vi "subDFD_REMEZ Spec Conversion.vi"(6 "fs [Hz]":dbl=1.0, 7 "Filter Type":T2(ring), 8 "f4 [Hz]":dbl, 9 "f3 [Hz]":dbl, 10 "f2 [Hz]":dbl=0.45, 11 "f1 [Hz]":dbl=0.12) -> (2 "band specs":T1(array[cluster])=[{"band specification"=[{"freq"=0.0, "amplitude"=1.0, "weight"=1.0}, {"freq"=0.2, "amplitude"=1.0, "weight"=1.0}], "ripple constraint"=0.0}, {"band specification"=[{"freq"=0.3, "amplitude"=0.0, "weight"=1.0}, {"freq"=0.5, "amplitude"=0.0, "weight"=1.0}], "ripple constraint"=0.0}])   [LabVIEW 2023]
panel:
  # "freq"
  # "amplitude"
  # "weight"
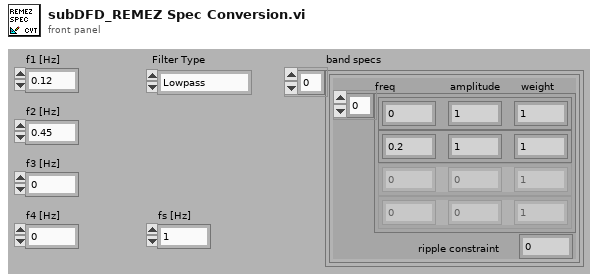
[diagram p1: front panel]
types:
  T1 = cluster{"band specification":cluster{"freq":dbl, "amplitude":dbl, "weight":dbl}[], "ripple constraint":dbl}[]
  T2 = enum16{"Lowpass", "Highpass", "Bandpass", "Bandstop"}
  T3 = cluster{cluster{"f2 [Hz]":dbl, dbl, dbl}[], dbl}[]
  T4 = cluster{cluster{"f4 [Hz]":dbl, dbl, dbl}[], dbl}[]
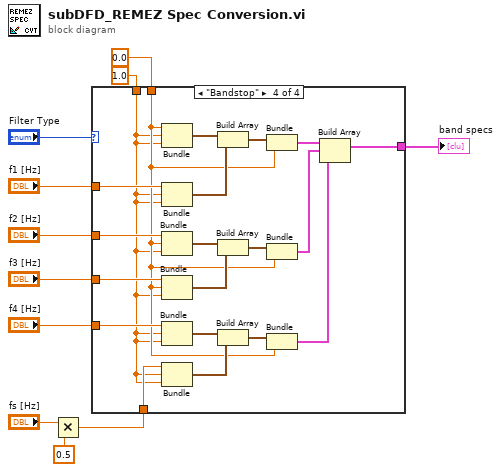
[diagram p0: block diagram]
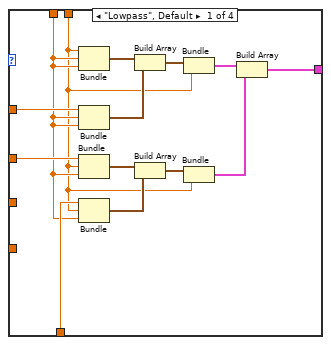
[diagram p2: hidden frame]
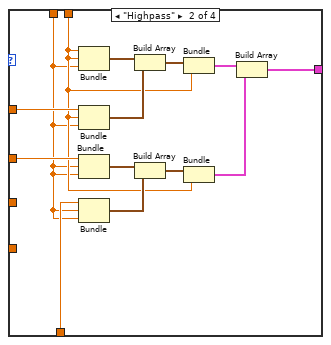
[diagram p3: hidden frame]
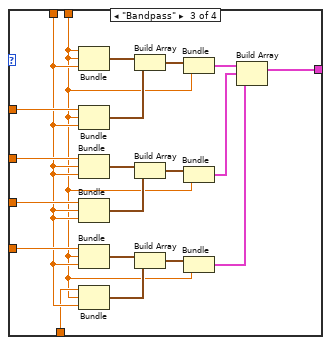
[diagram p4: hidden frame]
diagram:
  n1 = Multiply(x="fs [Hz]", y=0.5) -> (x*y=w4:dbl)
  n2 = case shown="\"Bandstop\"" "Filter Type" {
    tunnel: "f1 [Hz]" -> [w25 w39 w59 w79]
    tunnel: "f2 [Hz]" -> [w24 w38 w58 w78]
    tunnel: 0.0 -> [w15 w27 w42 w61]
    tunnel: 1.0 -> [w22 w26 w47 w60]
    tunnel: w4 -> [w23 w37 w46 w67]
    tunnel: [w12 w28 w40 w62] -> w3
    tunnel: "f3 [Hz]" -> [_ _ w49 w69]
    tunnel: "f4 [Hz]" -> [_ _ w48 w68]
    frame "Lowpass", Default {
      n3 = Bundle(w15, w22, w22) -> (w21:cluster{dbl, dbl, dbl})  [unwired: 1 out]
      n4 = Bundle("f1 [Hz]"=w25, w22, w22) -> (w20:cluster{"f1 [Hz]":dbl, dbl, dbl})  [unwired: 1 out]
      n5 = Bundle("f2 [Hz]"=w24, w15, w22) -> (w18:cluster{"f2 [Hz]":dbl, dbl, dbl})  [unwired: 1 out]
      n6 = Bundle(w23, w15, w22) -> (w17:cluster{dbl, dbl, dbl})  [unwired: 1 out]
      n7 = Build Array(w21, w20) -> (w19:cluster{"f1 [Hz]":dbl, dbl, dbl}[])
      n8 = Build Array(w18, w17) -> (w16:cluster{"f2 [Hz]":dbl, dbl, dbl}[])
      n9 = Bundle(w19, w15) -> (w14:cluster{cluster{"f1 [Hz]":dbl, dbl, dbl}[], dbl})  [unwired: 1 out]
      n10 = Bundle(w16, w15) -> (w13:cluster{cluster{"f2 [Hz]":dbl, dbl, dbl}[], dbl})  [unwired: 1 out]
      n11 = Build Array(w14, w13) -> (w12:T3)
    }
    frame "Highpass" {
      n12 = Bundle(w27, w27, w26) -> (w36:cluster{dbl, dbl, dbl})  [unwired: 1 out]
      n13 = Bundle("f1 [Hz]"=w39, w27, w26) -> (w35:cluster{"f1 [Hz]":dbl, dbl, dbl})  [unwired: 1 out]
      n14 = Bundle("f2 [Hz]"=w38, w26, w26) -> (w33:cluster{"f2 [Hz]":dbl, dbl, dbl})  [unwired: 1 out]
      n15 = Bundle(w37, w26, w26) -> (w32:cluster{dbl, dbl, dbl})  [unwired: 1 out]
      n16 = Build Array(w36, w35) -> (w34:cluster{"f1 [Hz]":dbl, dbl, dbl}[])
      n17 = Build Array(w33, w32) -> (w31:cluster{"f2 [Hz]":dbl, dbl, dbl}[])
      n18 = Bundle(w34, w27) -> (w30:cluster{cluster{"f1 [Hz]":dbl, dbl, dbl}[], dbl})  [unwired: 1 out]
      n19 = Bundle(w31, w27) -> (w29:cluster{cluster{"f2 [Hz]":dbl, dbl, dbl}[], dbl})  [unwired: 1 out]
      n20 = Build Array(w30, w29) -> (w28:T3)
    }
    frame "Bandpass" {
      n21 = Bundle(w42, w42, w47) -> (w57:cluster{dbl, dbl, dbl})  [unwired: 1 out]
      n22 = Bundle("f1 [Hz]"=w59, w42, w47) -> (w56:cluster{"f1 [Hz]":dbl, dbl, dbl})  [unwired: 1 out]
      n23 = Bundle("f2 [Hz]"=w58, w47, w47) -> (w54:cluster{"f2 [Hz]":dbl, dbl, dbl})  [unwired: 1 out]
      n24 = Bundle("f3 [Hz]"=w49, w47, w47) -> (w53:cluster{"f3 [Hz]":dbl, dbl, dbl})  [unwired: 1 out]
      n25 = Bundle("f4 [Hz]"=w48, w42, w47) -> (w45:cluster{"f4 [Hz]":dbl, dbl, dbl})  [unwired: 1 out]
      n26 = Bundle(w46, w42, w47) -> (w44:cluster{dbl, dbl, dbl})  [unwired: 1 out]
      n27 = Build Array(w57, w56) -> (w55:cluster{"f1 [Hz]":dbl, dbl, dbl}[])
      n28 = Build Array(w54, w53) -> (w52:cluster{"f3 [Hz]":dbl, dbl, dbl}[])
      n29 = Build Array(w45, w44) -> (w43:cluster{"f4 [Hz]":dbl, dbl, dbl}[])
      n30 = Bundle(w55, w42) -> (w51:cluster{cluster{"f1 [Hz]":dbl, dbl, dbl}[], dbl})  [unwired: 1 out]
      n31 = Bundle(w52, w42) -> (w50:cluster{cluster{"f3 [Hz]":dbl, dbl, dbl}[], dbl})  [unwired: 1 out]
      n32 = Bundle(w43, w42) -> (w41:cluster{cluster{"f4 [Hz]":dbl, dbl, dbl}[], dbl})  [unwired: 1 out]
      n33 = Build Array(w51, w50, w41) -> (w40:T4)
    }
    frame "Bandstop" {
      n34 = Bundle(w61, w60, w60) -> (w77:cluster{dbl, dbl, dbl})  [unwired: 1 out]
      n35 = Bundle("f1 [Hz]"=w79, w60, w60) -> (w76:cluster{"f1 [Hz]":dbl, dbl, dbl})  [unwired: 1 out]
      n36 = Bundle("f2 [Hz]"=w78, w61, w60) -> (w74:cluster{"f2 [Hz]":dbl, dbl, dbl})  [unwired: 1 out]
      n37 = Bundle("f3 [Hz]"=w69, w61, w60) -> (w73:cluster{"f3 [Hz]":dbl, dbl, dbl})  [unwired: 1 out]
      n38 = Bundle("f4 [Hz]"=w68, w60, w60) -> (w66:cluster{"f4 [Hz]":dbl, dbl, dbl})  [unwired: 1 out]
      n39 = Bundle(w67, w60, w60) -> (w65:cluster{dbl, dbl, dbl})  [unwired: 1 out]
      n40 = Build Array(w77, w76) -> (w75:cluster{"f1 [Hz]":dbl, dbl, dbl}[])
      n41 = Build Array(w74, w73) -> (w72:cluster{"f3 [Hz]":dbl, dbl, dbl}[])
      n42 = Build Array(w66, w65) -> (w64:cluster{"f4 [Hz]":dbl, dbl, dbl}[])
      n43 = Bundle(w75, w61) -> (w71:cluster{cluster{"f1 [Hz]":dbl, dbl, dbl}[], dbl})  [unwired: 1 out]
      n44 = Bundle(w72, w61) -> (w70:cluster{cluster{"f3 [Hz]":dbl, dbl, dbl}[], dbl})  [unwired: 1 out]
      n45 = Bundle(w64, w61) -> (w63:cluster{cluster{"f4 [Hz]":dbl, dbl, dbl}[], dbl})  [unwired: 1 out]
      n46 = Build Array(w71, w70, w63) -> (w62:T4)
    }
  }
  "band specs" <- w3
